vi "DataQA.vi"(1 "Quality cuts":bool, 2 "Data In":dbl[](array[numeric])) -> (0 "Data Out":dbl[](array[numeric]))   [LabVIEW 2018]
uses:
  <vilib>/Analysis/NI_AALBase.lvlib
panel:
  # "Makes qualiy cuts on data"
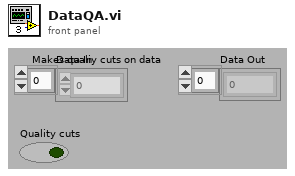
[diagram p1: front panel]
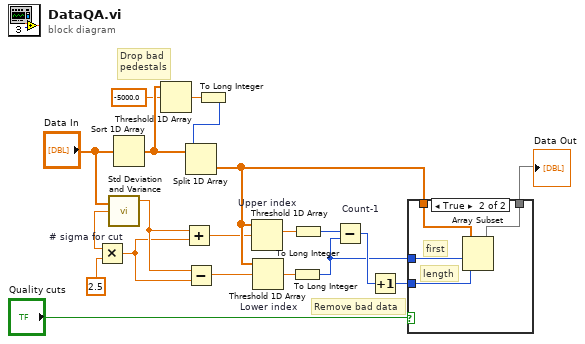
[diagram p0: block diagram]
diagram:
  # "Remove bad data"
  # "Drop bad\npedestals"
  n1 = call <vilib>:"Std Deviation and Variance.vi"("X"="Data In") -> ("mean"=w4:dbl, "standard deviation"=w5:dbl)  [unwired: 1 in, 1 out]
  n2 = Multiply "# sigma for cut"(x=w5, y=2.5) -> (x*y=w1:dbl)
  n3 = Sort 1D Array(array="Data In") -> (sorted array=w14:dbl[])
  n4 = Threshold 1D Array(2:-5000.0, 3:w14) -> (0:w19:dbl)  [unwired: 1 in]
  n5 = Add(x=w4, y=w1) -> (x+y=w2:dbl)
  n6 = Subtract(x=w4, y=w1) -> (x-y=w3:dbl)
  n7 = To Long Integer(number=w19) -> (32bit integer=w12:i32)
  n8 = Split 1D Array(array=w14, index=w12) -> (second subarray=w15:dbl[])  [unwired: 1 out]
  n9 = Threshold 1D Array "Upper index"(2:w2, 3:w15) -> (0:w7:dbl)  [unwired: 1 in]
  n10 = Threshold 1D Array "Lower index"(2:w3, 3:w15) -> (0:w20:dbl)  [unwired: 1 in]
  n11 = To Long Integer(number=w20) -> (32bit integer=w8:i32)
  n12 = To Long Integer(number=w7) -> (32bit integer=w6:i32)
  n13 = Subtract "Count-1"(x=w6, y=w8) -> (x-y=w9:i32)
  n14 = Increment(x=w9) -> (x+1=w10:i32)
  n15 = case shown="True" "Quality cuts" {
    tunnel: w8 -> [_ w25]
    tunnel: w10 -> [_ w24]
    tunnel: [w21 w23] -> w18
    tunnel: w15 -> [w21 w22]
    frame False {
    }
    frame True {
      # "length"
      # "first"
      n16 = Array Subset "Array Subset"(array=w22, index=w25, length=w24) -> (w23:dbl[])
    }
  }
  "Data Out" <- w18
